vi "Main.vi"(8 "error in (no error)":errorcluster, 11 "Process in":refnum<class "Output Process.lvclass">) -> (0 "error out":errorcluster, 3 "Process out":refnum<class "Output Process.lvclass">)   [LabVIEW 2019, in "TimingDRV Engine.lvlib" / "Output Process.lvclass"]
uses:
  Output Process.lvclass
  C:/Users/XEnderMD/Desktop/CD Project Tools/Source/Engine/Parent Classes/Process/Process.lvclass
  ee6b0e45-0e4e-4b42-bcc4-620819e24e27.vi
  Parent Classes/Process/Process.lvclass
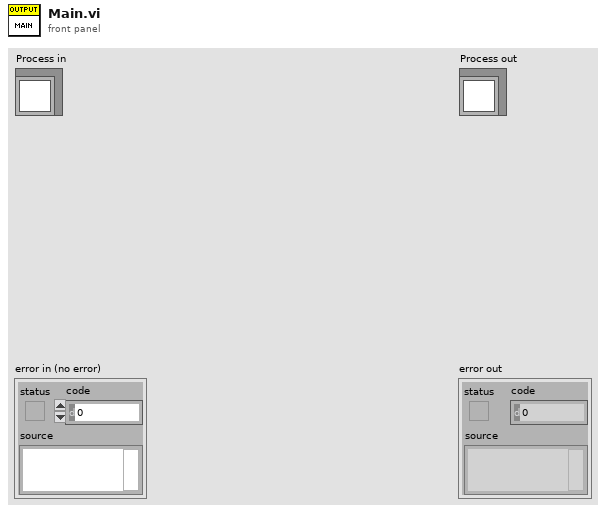
[diagram p1: front panel]
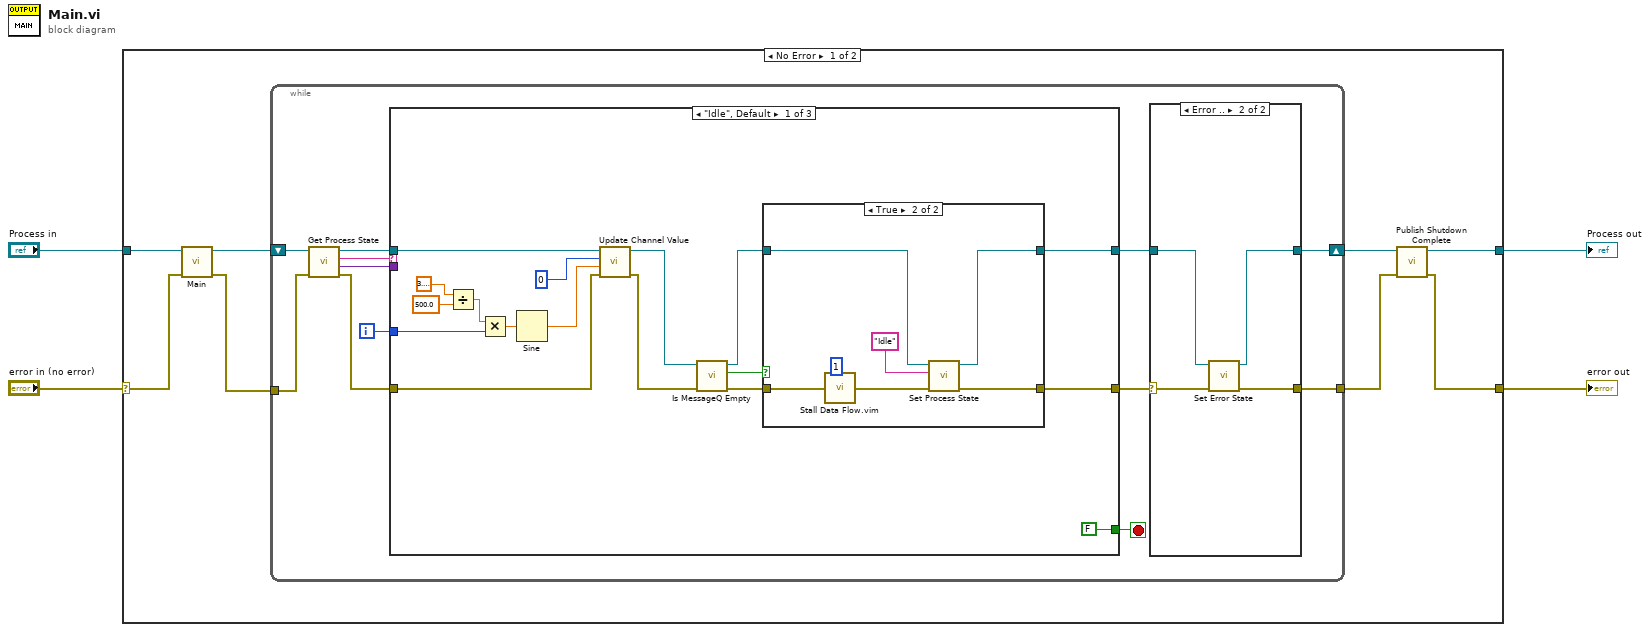
[diagram p0: block diagram]
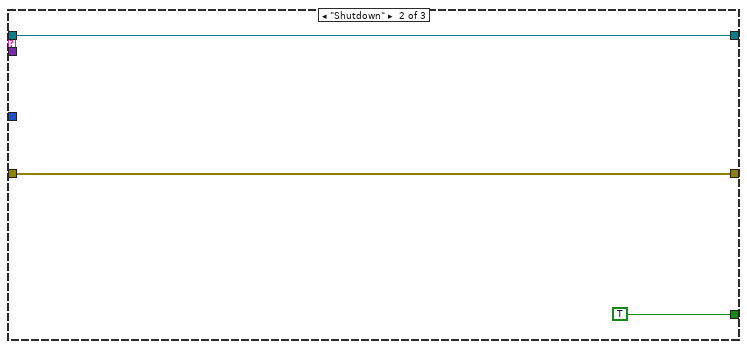
[diagram p4: hidden frame]
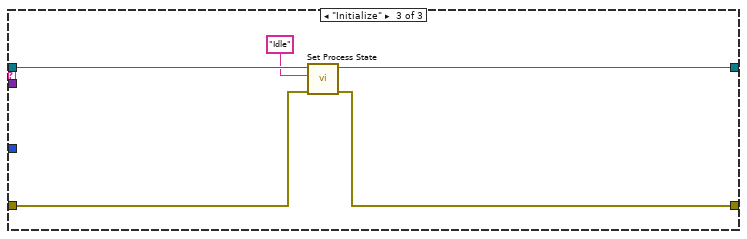
[diagram p5: hidden frame]
diagram:
  n1 = case shown="No Error" "error in (no error)" {
    selector: "error in (no error)" -> [w11 w66]
    tunnel: [w5 w66] -> w1
    tunnel: [w7 w65] -> w2
    tunnel: "Process in" -> [w12 w65]
    frame No Error {
      n2 = call-parent "Main.vi"("error in (no error)"=w11, "Process in"=w12) -> ("error out"=w9:errorcluster, "Process out"=w10:refnum<class "Output Process.lvclass">)  [unwired: 8 in]
      n3 = while {
        shift-right: [w17] -> w8
        shift-left: w10 -> [w23]
        tunnel: w9 -> [w24]
        tunnel: [w16] -> w6
        i -> [w13]
        stop <- w15 stop-if-true
        n4 = call "Get Process State.vi"("error in (no error)"=w24, "Process in"=w23) -> ("error out"=w20:errorcluster, "Payload"=w21:variant, "Command"=w14:string, "Process out"=w22:refnum<class "Output Process.lvclass">)  [unwired: 6 in]
        n5 = case shown="\"Idle\", Default" w14 {
          tunnel: w22 -> [w46 w59 w64]
          tunnel: w21 -> [_ _ _]
          tunnel: w20 -> [w45 w58 w63]
          tunnel: [w38 w59 w62] -> w19
          tunnel: [w37 w58 w61] -> w18
          tunnel: [FALSE TRUE _] -> w15
          tunnel: w13 -> [w34 _ _]
          frame "Idle", Default {
            n6 = Divide(x=3.141592653589793, y=500.0) -> (x/y=w33:dbl)
            n7 = Multiply(x=w33, y=w34) -> (x*y=w32:dbl)
            n8 = Sine(x=w32) -> (sin(x)=w31:dbl)
            n9 = call "Update Channel Value.vi"("error in (no error)"=w45, "New Value"=w31, "Channel Index"=0, "Output Process in"=w46) -> ("error out"=w43:errorcluster, "Output Process out"=w42:refnum<class "Output Process.lvclass">)  [unwired: 4 in, 2 out]
            n10 = call "Is MessageQ Empty.vi"("error in (no error)"=w43, "Process in"=w42) -> ("error out"=w40:errorcluster, "is Empty ?"=w41:bool, "Process out"=w39:refnum<class "Output Process.lvclass">)  [unwired: 7 in]
            n11 = case shown="True" w41 {
              tunnel: w40 -> [w48 w52]
              tunnel: w39 -> [w49 w55]
              tunnel: [w49 w54] -> w38
              tunnel: [w48 w53] -> w37
              frame False {
              }
              frame True {
                n12 = call "Stall Data Flow.vim"("value in"=w52, "milliseconds to wait"=u32 1) -> ("value out"=w51:errorcluster)  [unwired: 1 out]
                n13 = call "Set Process State.vi"("error in (no error)"=w51, "Command"="Idle", "Process in"=w55) -> ("error out"=w53:errorcluster, "Process out"=w54:refnum<class "Output Process.lvclass">)  [unwired: 7 in]
              }
            }
          }
          frame "Shutdown" {
          }
          frame "Initialize" {
            n14 = call "Set Process State.vi"("error in (no error)"=w63, "Command"="Idle", "Process in"=w64) -> ("error out"=w61:errorcluster, "Process out"=w62:refnum<class "Output Process.lvclass">)  [unwired: 7 in]
          }
        }
        n15 = case shown="Error .." w18 {
          selector: w18 -> [w25 w30]
          tunnel: w19 -> [w26 w29]
          tunnel: [w26 w28] -> w17
          tunnel: [w25 w27] -> w16
          frame No Error {
          }
          frame Error {
            n16 = call "Set Error State.vi"("error in (no error)"=w30, "Process in"=w29) -> ("error out"=w27:errorcluster, "Process out"=w28:refnum<class "Output Process.lvclass">)  [unwired: 8 in]
          }
        }
      }
      n17 = call "Publish Shutdown Complete.vi"("error in (no error)"=w6, "Process in"=w8) -> ("error out"=w5:errorcluster, "Process out"=w7:refnum<class "Output Process.lvclass">)  [unwired: 8 in]
    }
    frame Error {
    }
  }
  "error out" <- w1
  "Process out" <- w2
